vi "Keithley DMM6500 DAQ6500 Series Digitizing to Obtain Average Current.vi"() -> ()   [LabVIEW 2015]
doc: "This example shows how to obtain the average current."
uses:
  <instrlib>/Keithley DMM6500 DAQ6500 Series/Keithley DMM6500 DAQ6500 Series.lvlib
panel:
  out "Average Current":dbl
  out "Actual Readings":i32
  out "Full Output Data Path":path
  out "Output File Name":string
  in  "Data Extraction Size (100)":i32=100
  out "Measurements":sgl[](array[numeric])
  in  "Manual Range (1)":dbl=1.0
  in  "Buffer Name (\"digiBuff\")":string="digiBuff"
  in  "Count (1E+5)":u32=100000
  in  "Sample Rate (1E+6)":dbl=1000000.0
  in  "Function (14: Digitize Current)":i32(ring)=14 items=["Digitize Voltage"=13, "Digitize Current"=14]
  in  "VISA resource name":refnum<visa-resource-name>
  # "(c) 2019 - 2022 National Instruments.  ALL RIGHTS RESERVED."
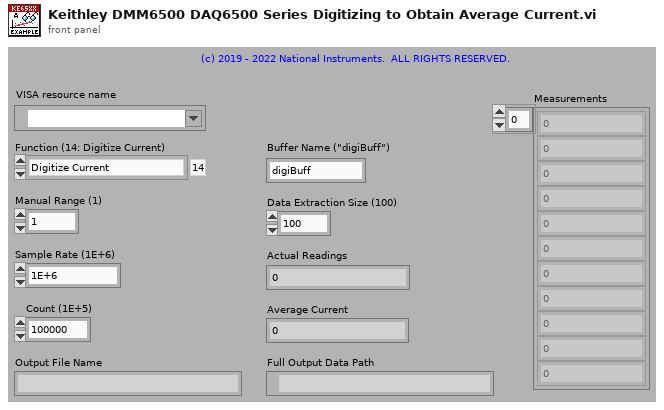
[diagram p1: front panel]
types:
  T1 = enum16{"open", "replace", "create", "open or create", "replace or create", "replace or create with confirmation"}
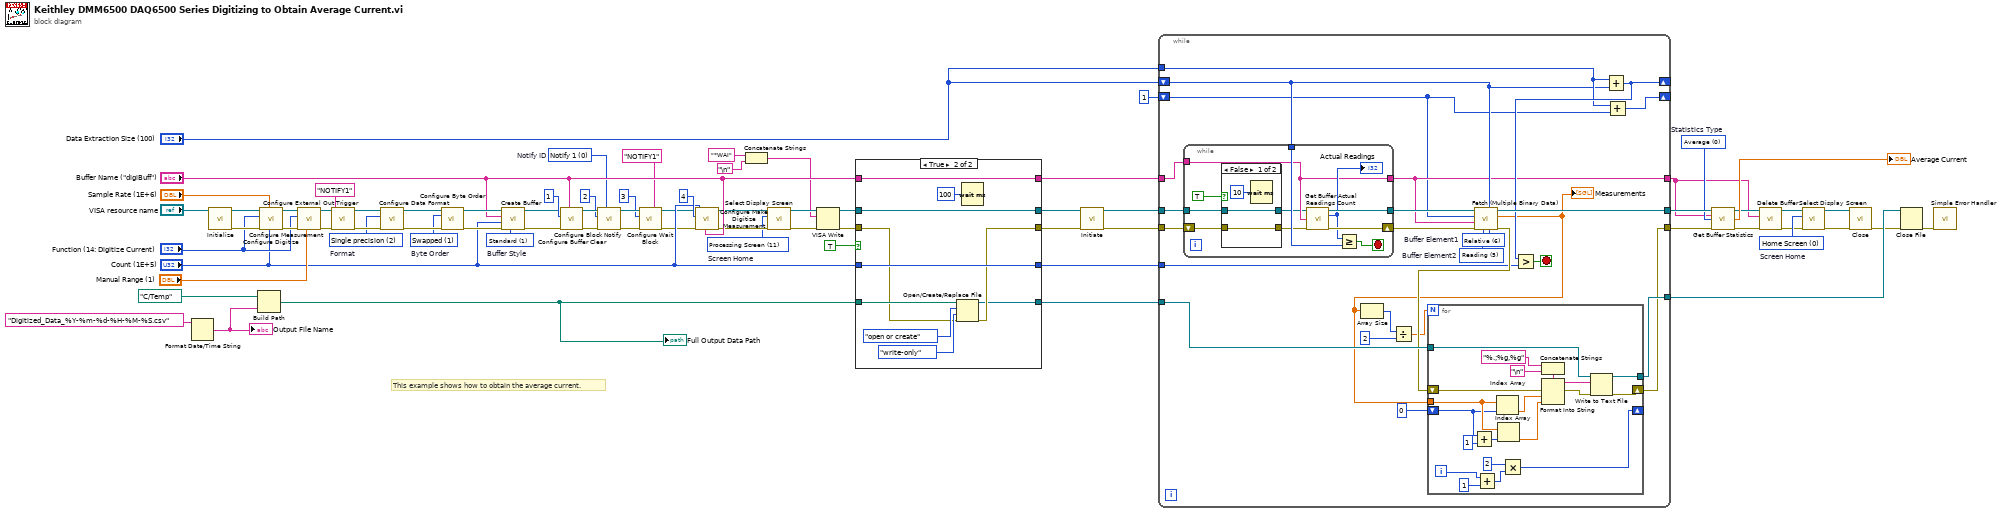
[diagram p0: block diagram]
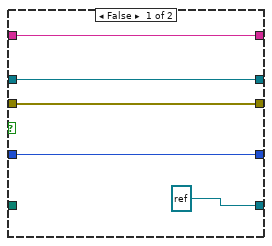
[diagram p2: hidden frame]
diagram:
  w7 = 0 items=["Average", "Maximum", "Minimum", "Peak-to-peak", "Standard deviation"]  # Statistics Type
  w20 = 0 items=["Notify 1", "Notify 2", "Notify 3", "Notify 4", "Notify 5", "Notify 6", "Notify 7", "Notify 8"]  # Notify ID
  w37 = u16 0 items=["Home Screen", "Home Large Reading", "Reading Sheet", "Graph Screen", "Histogram", "Functions Swipe", "Graph Swipe", "Secondary Swipe", "Settings Swipe", "Statistics Swipe", "User Swipe", "Processing Screen"]  # Screen Home
  w40 = u16 11 items=["Home Screen", "Home Large Reading", "Reading Sheet", "Graph Screen", "Histogram", "Functions Swipe", "Graph Swipe", "Secondary Swipe", "Settings Swipe", "Statistics Swipe", "User Swipe", "Processing Screen"]  # Screen Home
  w58 = u16 1 items=["Normal", "Swapped"]  # Byte Order
  w1 = u16 2 items=["ASCII", "Double precision", "Single precision"]  # Format
  w63 = 1 items=["Compact", "Standard", "Full", "Writable", "Full Writable"]  # Buffer Style
  # "This example shows how to obtain the average current."
  n1 = Format Date/Time String(time format string (%c)="Digitized_Data_%Y-%m-%d-%H-%M-%S.csv") -> (date/time string=w44:string)  [unwired: 2 in]
  "Output File Name" <- w44
  n2 = call <instrlib>:"Initialize.vi"("VISA resource name"="VISA resource name") -> ("error out"=w73:errorcluster, "VISA resource name out"=w72:refnum<visa-resource-name>)  [unwired: 9 in]
  n3 = Build Path(base path=path "C:/Temp" ("file path (use dialog)"), name or relative path=w44) -> (appended path=w43:path)
  "Full Output Data Path" <- w43
  n4 = call <instrlib>:"Configure Digitize.vi"("Count (1)"="Count (1E+5)", "Sample Rate (1E+6)"="Sample Rate (1E+6)", "error in (no error)"=w73, "Function (13: Digitize Voltage)"="Function (14: Digitize Current)", "VISA resource name"=w72) -> ("error out"=w70:errorcluster, "VISA resource name out"=w71:refnum<visa-resource-name>)  [unwired: 5 in]
  n5 = call <instrlib>:"Configure Measurement.vi"("Manual Range (1)"="Manual Range (1)", "error in (no error)"=w70, "Function (0: Voltage DC)"="Function (14: Digitize Current)", "VISA resource name"=w71) -> ("error out"=w24:errorcluster, "VISA resource name out"=w25:refnum<visa-resource-name>)  [unwired: 6 in]
  n6 = call <instrlib>:"Configure External Out Trigger.vi"("error in (no error)"=w24, "External Stimulus Event (\"NONE\")"="NOTIFY1" ("External Stimulus Event (\"NONE\")"), "VISA resource name"=w25) -> ("error out"=w22:errorcluster, "VISA resource name out"=w23:refnum<visa-resource-name>)  [unwired: 7 in]
  n7 = call <instrlib>:"Configure Data Format.vi"("error in (no error)"=w22, "Format (0: ASCII)"=w1, "VISA resource name"=w23) -> ("error out"=w61:errorcluster, "VISA resource name out"=w62:refnum<visa-resource-name>)  [unwired: 7 in]
  n8 = call <instrlib>:"Configure Byte Order.vi"("VISA resource name"=w62, "Byte Order"=w58, "error in (no error)"=w61) -> ("VISA resource name out"=w60:refnum<visa-resource-name>, "error out"=w59:errorcluster)  [unwired: 11 in]
  n9 = call <instrlib>:"Create Buffer.vi"("Buffer Style (1: Standard)"=w63, "error in (no error)"=w59, "Buffer Size (10)"="Count (1E+5)", "Buffer Name (\"\")"="Buffer Name (\"digiBuff\")", "VISA resource name"=w60) -> ("error out"=w65:errorcluster, "VISA resource name out"=w64:refnum<visa-resource-name>)  [unwired: 5 in]
  n10 = call <instrlib>:"Configure Buffer Clear.vi"("Buffer Name (\"\")"="Buffer Name (\"digiBuff\")", "error in (no error)"=w65, "Block Number (1)"=u32 1 ("Block Number (0)"), "VISA resource name"=w64) -> ("error out"=w18:errorcluster, "VISA resource name out"=w19:refnum<visa-resource-name>)  [unwired: 6 in]
  n11 = call <instrlib>:"Configure Block Notify.vi"("Notify ID (0: Notify 1)"=w20, "error in (no error)"=w18, "Block Number (1)"=u32 2 ("Block Number (0)"), "VISA resource name"=w19) -> ("error out"=w16:errorcluster, "VISA resource name out"=w15:refnum<visa-resource-name>)  [unwired: 6 in]
  n12 = call <instrlib>:"Configure Wait Block.vi"("Event1 (\"\")"="NOTIFY1" ("Event1 (\"\")"), "error in (no error)"=w16, "Block Number (1)"=u32 3 ("Block Number (0)"), "VISA resource name"=w15) -> ("error out"=w12:errorcluster, "VISA resource name out"=w11:refnum<visa-resource-name>)  [unwired: 6 in]
  n13 = call <instrlib>:"Configure Make Digitize Measurement.vi"("Buffer Name (\"defbuffer1\")"="Buffer Name (\"digiBuff\")", "error in (no error)"=w12, "Readings Count (1)"="Count (1E+5)", "Block Number (1)"=u32 4 ("Block Number (0)"), "VISA resource name"=w11) -> ("error out"=w41:errorcluster, "VISA resource name out"=w42:refnum<visa-resource-name>)  [unwired: 5 in]
  n14 = Concatenate Strings("*WAI" ("write buffer"), "\n") -> (w26:string)
  n15 = call <instrlib>:"Select Display Screen.vi"("error in (no error)"=w41, "Screen Home"=w40, "VISA resource name"=w42) -> ("error out"=w35:errorcluster, "VISA resource name out"=w36:refnum<visa-resource-name>)  [unwired: 7 in]
  n16 = VISA Write(VISA resource name=w36, write buffer=w26, error in (no error)=w35) -> (VISA resource name out=w33:refnum<visa-resource-name>, error out=w31:errorcluster)  [unwired: 1 out]
  n17 = case shown="True" TRUE {
    tunnel: w33 -> [w79 w90]
    tunnel: w31 -> [w78 w81]
    tunnel: [w79 w90] -> w34
    tunnel: [w78 w86] -> w32
    tunnel: "Count (1E+5)" -> [w77 w88]
    tunnel: "Buffer Name (\"digiBuff\")" -> [w80 w89]
    tunnel: [w80 w89] -> w52
    tunnel: [w77 w88] -> w53
    tunnel: w43 -> [_ w82]
    tunnel: [refnum<file> refnum ("refnum out") w85] -> w50
    frame False {
    }
    frame True {
      n18 = Open/Create/Replace File(file path (use dialog)=w82, error in=w81, operation (0:open)=T1."open or create", access (0:read/write)=enum16{"read/write", "read-only", "write-only"}."write-only") -> (refnum out=w85:refnum<file>, error out=w86:errorcluster)  [unwired: 2 in, 1 out]
      n19 = Wait (ms)(milliseconds to wait=u32 100) -> ()  [unwired: 1 out]
    }
  }
  n20 = call <instrlib>:"Initiate.vi"("error in (no error)"=w32, "VISA resource name"=w34) -> ("error out"=w29:errorcluster, "VISA resource name out"=w30:refnum<visa-resource-name>)  [unwired: 8 in]
  n21 = while {
    shift-right: [w113] -> _
    shift-left: 1 ("Start Index (1)") -> [w91]
    shift-right: [w111] -> _
    shift-left: "Data Extraction Size (100)" -> [w94]
    tunnel: "Data Extraction Size (100)" -> [w99]
    tunnel: w30 -> [w98]
    tunnel: w29 -> [w97]
    tunnel: w52 -> [w93]
    tunnel: [w114] -> w10
    tunnel: [w106] -> w9
    tunnel: [w92] -> w2
    tunnel: w53 -> [w100]
    tunnel: w50 -> [w109]
    tunnel: [w108] -> w49
    stop <- w112 stop-if-true
    w110 = 5 items=["", "Date", "Extra", "Formatted", "Fractional", "Reading", "Relative", "Seconds", "Status", "Time", "Tstamp", "Unit", "CHAN", "Extra Form", "Extra Unit"]  # Buffer Element2
    w115 = 6 items=["", "Date", "Extra", "Formatted", "Fractional", "Reading", "Relative", "Seconds", "Status", "Time", "Tstamp", "Unit", "CHAN", "Extra Format", "Extra Unit"]  # Buffer Element1
    n22 = while {
      tunnel: w93 -> [w121]
      shift-right: [w125] -> w95
      shift-left: w97 -> [w120]
      tunnel: w94 -> [w122]
      tunnel: w98 -> [w118]
      tunnel: [w126] -> w96
      tunnel: [w121] -> w92
      stop <- w124 stop-if-true
      n23 = case shown="False" TRUE {
        tunnel: w120 -> [w128 w131]
        tunnel: [w128 w131] -> w119
        tunnel: w118 -> [w129 w130]
        tunnel: [w129 w130] -> w117
        frame False {
          n24 = Wait (ms)(milliseconds to wait=u32 10) -> ()  [unwired: 1 out]
        }
        frame True {
        }
      }
      n25 = call <instrlib>:"Get Buffer Actual Readings Count.vi"("VISA resource name"=w117, "Buffer Name (defbuffer1)"=w121, "error in (no error)"=w119) -> ("VISA resource name out"=w126:refnum<visa-resource-name>, "Actual Readings"=w123:i32, "error out"=w125:errorcluster)  [unwired: 10 in]
      "Actual Readings" <- w123
      n26 = Greater Or Equal?(x=w123, y=w122) -> (x >= y?=w124:bool)
    }
    n27 = call <instrlib>:"Fetch (Multiple Binary Data).vi"("Buffer Element2"=w110, "End Index (10)"=w94, "Buffer Element1"=w115, "error in (no error)"=w95, "Buffer Name"=w92, "Start Index (1)"=w91, "VISA resource name"=w96) -> ("error out"=w107:errorcluster, "Measurements"=w105:sgl[], "VISA resource name out"=w114:refnum<visa-resource-name>)  [unwired: 2 in]
    "Measurements" <- w105
    n28 = Array Size(array=w105) -> (size(s)=w103:i32)
    n29 = Divide(x=w103, y=2 ("x")) -> (x/y=w101:dbl)
    n30 = for {
      N: w101 -> [_]
      shift-right: [w144] -> w106
      shift-left: w107 -> [w145]
      tunnel: w105 -> [w143]
      tunnel: w109 -> [w151]
      tunnel: [w150] -> w108
      shift-right: [w134] -> _
      shift-left: 0 ("index") -> [w135]
      i -> [w136]
      n31 = Add(x=w135, y=1) -> (x+y=w139:i32)
      n32 = Add(x=w136, y=1) -> (x+y=w137:i32)
      n33 = Index Array(array=w143, index=w135) -> (element=w142:sgl)
      n34 = Index Array(array=w143, index=w139) -> (element=w141:sgl)
      n35 = Multiply(x=2, y=w137) -> (x*y=w134:i32)
      n36 = Concatenate Strings("%.;%g,%g" ("format string"), "\n") -> (w146:string)
      n37 = Format Into String(format string=w146, error in=w145, w142, w141) -> (resulting string=w133:string, error out=w149:errorcluster)  [unwired: 1 in]
      n38 = Write to Text File(file (use dialog)=w151, text=w133, error in=w149) -> (refnum out=w150:refnum<file>, error out=w144:errorcluster)  [unwired: 1 in, 1 out]
    }
    n39 = Add(x=w99, y=w94) -> (x+y=w111:i32)
    n40 = Greater?(x=w111, y=w100) -> (0:w112:bool)
    n41 = Add(x=w99, y=w91) -> (x+y=w113:i32)
  }
  n42 = call <instrlib>:"Get Buffer Statistics.vi"("VISA resource name"=w10, "Buffer Name (defbuffer1)"=w2, "Statistics Type"=w7, "error in (no error)"=w9) -> ("VISA resource name out"=w6:refnum<visa-resource-name>, "Statistics Value"=→"Average Current":dbl, "error out"=w5:errorcluster)  [unwired: 9 in]
  n43 = call <instrlib>:"Delete Buffer.vi"("error in (no error)"=w5, "Buffer Name (\"\")"=w2, "VISA resource name"=w6) -> ("error out"=w3:errorcluster, "VISA resource name out"=w4:refnum<visa-resource-name>)  [unwired: 7 in]
  n44 = call <instrlib>:"Select Display Screen.vi"("error in (no error)"=w3, "Screen Home"=w37, "VISA resource name"=w4) -> ("error out"=w39:errorcluster, "VISA resource name out"=w38:refnum<visa-resource-name>)  [unwired: 7 in]
  n45 = call <instrlib>:"Close.vi"("error in (no error)"=w39, "VISA resource name"=w38) -> ("error out"=w48:errorcluster)  [unwired: 9 in]
  n46 = Close File(refnum=w49, error in=w48) -> (error out=w47:errorcluster)  [unwired: 1 out]
  n47 = call <vilib>:"Simple Error Handler.vi"("error in (no error)"=w47) -> ()  [unwired: 4 in, 5 out]
